vi "Configure Pattern Trigger Source.vi"(8 "error in (no error)":errorcluster, 9 "BNC Connector (0: BB TRIG 1)":i32(ring) items=["BBTrigger1", "BBTrigger2", "Event1", "PTrigger", "No Pattern Trigger"], 10 "Pattern Trigger (1: Pattern Trigger 1)":i32(ring)=1 items=["Pattern Trigger 1"=1, "Pattern Trigger 2"=2], 11 "VISA resource name":refnum<visa-resource-name>) -> (0 "error out":errorcluster, 3 "VISA resource name out":refnum<visa-resource-name>)   [LabVIEW 2012, in "Agilent PSG MXG Series.lvlib"]
doc: "Selects a BNC connector to use as an input for the Pattern Trigger In source.\n\n<B>Notes:</B>\n(1) This VI is valid only in N5172B, N5182B.\n\n(2) For N5172B, this VI is valid only when the instrument installs <B>Option 653</B> or <B>Option 655</B>.\n\n(3) For N5182B, this VI is valid only when the instrument installs <B>Option 656</B> or <B>Option 657</B>."
uses:
  <instrlib>/Agilent PSG MXG Series/Agilent PSG MXG Series.lvlib
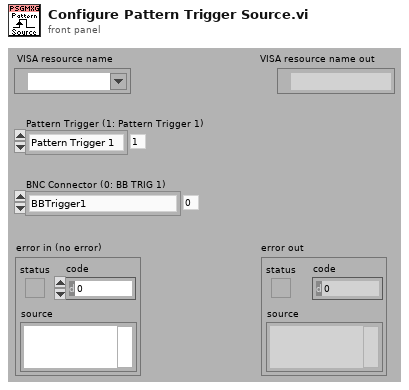
[diagram p1: front panel]
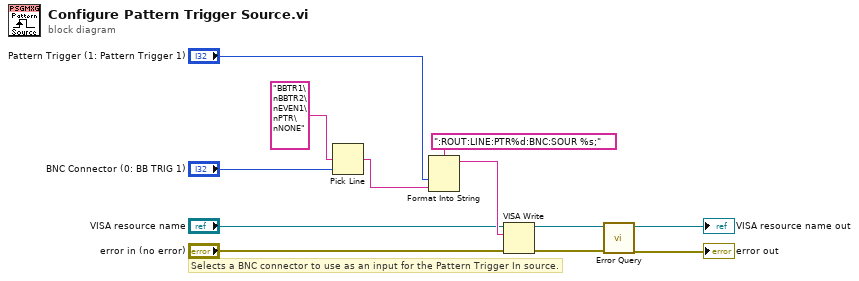
[diagram p0: block diagram]
diagram:
  # "Selects a BNC connector to use as an input for the Pattern Trigger In source."
  n1 = Pick Line(multi-line string="BBTR1\nBBTR2\nEVEN1\nPTR\nNONE", line index="BNC Connector (0: BB TRIG 1)") -> (output string=w8:string)  [unwired: 1 out]
  n2 = Format Into String(format string=":ROUT:LINE:PTR%d:BNC:SOUR %s;", "Pattern Trigger (1: Pattern Trigger 1)", w8) -> (resulting string=w7:string)  [unwired: 2 in, 1 out]
  n3 = VISA Write(VISA resource name="VISA resource name", write buffer=w7, error in (no error)="error in (no error)") -> (VISA resource name out=w4:refnum<visa-resource-name>, error out=w3:errorcluster)  [unwired: 1 out]
  n4 = call <instrlib>:"Error Query.vi"("error in (no error)"=w3, "VISA resource name"=w4) -> ("error out"=→"error out":errorcluster, "VISA resource name out"=→"VISA resource name out":refnum<visa-resource-name>)  [unwired: 8 out]
